vi "parseStatus.vi"(8 "error in (no error)":errorcluster, 10 "response":string, 11 "PlainTextResponseParser in":refnum<class "PlainTextResponseParser.lvclass">) -> (0 "error out":errorcluster, 2 "status":string, 3 "PlainTextResponseParser out":refnum<class "PlainTextResponseParser.lvclass">)   [LabVIEW 2023, in "AbstractFactory.lvlib" / "PlainTextResponseParser.lvclass"]
uses:
  PlainTextResponseParser.lvclass
  <vilib>/Utility/error.llb/Trim Whitespace One-Sided.vi
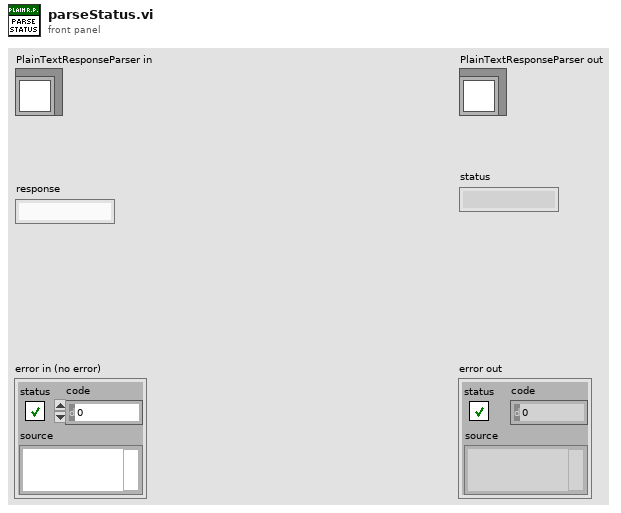
[diagram p1: front panel]
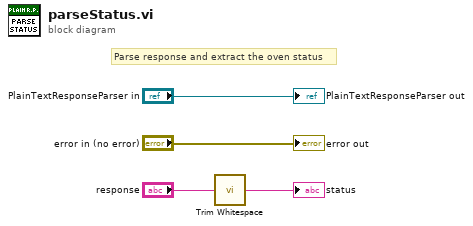
[diagram p0: block diagram]
diagram:
  # "Parse response and extract the oven status"
  n1 = call <vilib>:"Trim Whitespace.vi"("string"="response") -> ("trimmed string"=→"status":string)  [unwired: 1 in]
  "error out" <- "error in (no error)"
  "PlainTextResponseParser out" <- "PlainTextResponseParser in"
